vi "Add Cube.vi"(8 "error in (no error)":errorcluster, 10 "Cube":refnum<class "Cube.lvclass">, 11 "Cubes in":refnum<class "Cubes.lvclass">) -> (0 "error out":errorcluster, 3 "Cubes out":refnum<class "Cubes.lvclass">)   [LabVIEW 2019, in "22.lvlib" / "Cubes.lvclass"]
uses:
  Cubes.lvclass
  Cube/Cube.lvclass
  Cubes.lvclass/Cubes.ctl
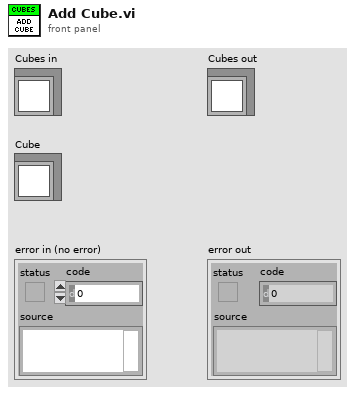
[diagram p1: front panel]
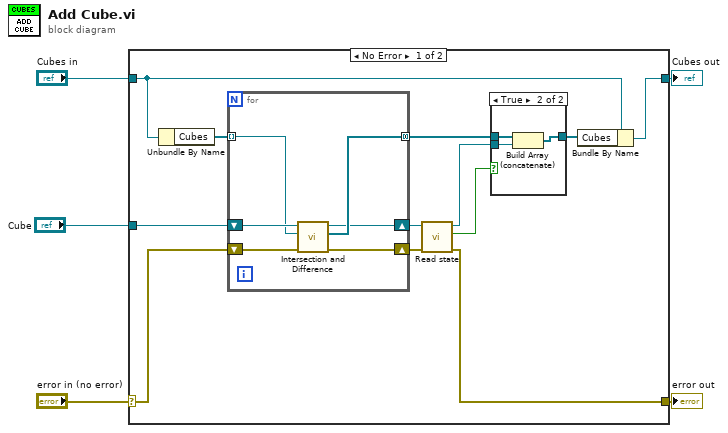
[diagram p0: block diagram]
diagram:
  n1 = case shown="No Error" "error in (no error)" {
    selector: "error in (no error)" -> [w7 w29]
    tunnel: [w6 w29] -> w4
    tunnel: [w16 w28] -> w2
    tunnel: "Cubes in" -> [w17 w28]
    tunnel: "Cube" -> [w8 _]
    frame No Error {
      n2 = Unbundle By Name(w17) -> ("Cubes"=w9:refnum<class "Cube.lvclass">[])
      n3 = for {
        tunnel: w9 -> [w26] mode=indexing
        tunnel: [w25] -> w12 mode=concatenating
        shift-right: [w23] -> w14
        shift-left: w7 -> [w24]
        shift-right: [w22] -> w15
        shift-left: w8 -> [w27]
        n4 = call-dynamic "Intersection and Difference.vi"("error in (no error)"=w24, "Cube A"=w26, "Cube B in"=w27) -> ("error out"=w23:errorcluster, "Difference"=w25:refnum<class "Cube.lvclass">[], "Cube B out"=w22:refnum<class "Cube.lvclass">)  [unwired: 4 in, 2 out]
      }
      n5 = call-dynamic "Read state.vi"("error in (no error)"=w14, "Cube in"=w15) -> ("error out"=w6:errorcluster, "state"=w13:bool, "Cube out"=w11:refnum<class "Cube.lvclass">)  [unwired: 7 in]
      n6 = case shown="True" w13 {
        tunnel: w12 -> [w18 w21]
        tunnel: [w18 w20] -> w10
        tunnel: w11 -> [_ w19]
        frame False {
        }
        frame True {
          n7 = Build Array (concatenate)(w21, w19) -> (w20:refnum<class "Cube.lvclass">[])
        }
      }
      n8 = Bundle By Name(cluster=w17, "Cubes"=w10) -> (w16:refnum<class "Cubes.lvclass">)
    }
    frame Error {
    }
  }
  "error out" <- w4
  "Cubes out" <- w2
